vi "Test Periodic Timing.vi"() -> ()   [LabVIEW 2023, in "Volatus.lvlib" / "Module.lvclass"]
uses:
  Module.lvclass
  Module.lvclass/Module.ctl
panel:
  out "XY Graph":cluster{"elements":dbl[], "elements":dbl[]}(graph)
  out "Deadline":u32
  out "Message":string
  out "Periodic":bool
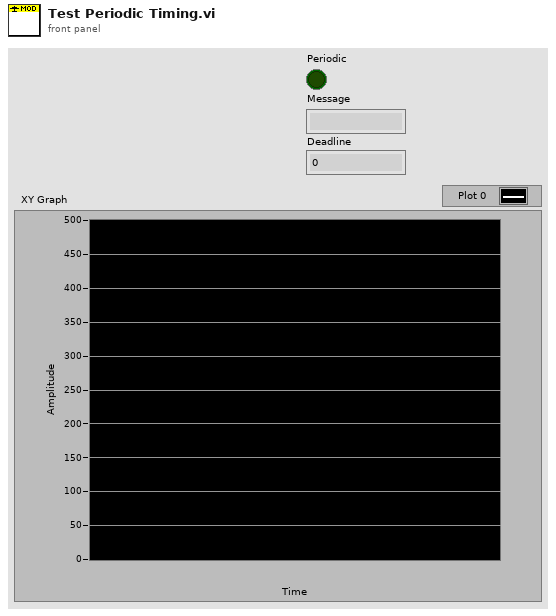
[diagram p1: front panel]
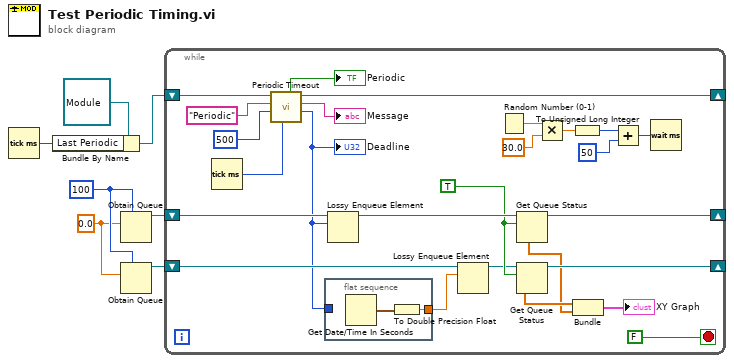
[diagram p0: block diagram]
diagram:
  w4 = 100 ("max queue size (-1, unlimited)")
  w3 = 0.0
  n1 = Tick Count (ms)() -> (millisecond timer value=w5:u32)
  n2 = Bundle By Name(cluster=refnum<class "Module.lvclass"> refnum ("Module in"), "Last Periodic"=w5) -> (w6:refnum<class "Module.lvclass">)
  n3 = Obtain Queue(max queue size (-1, unlimited)=w4, element data type=w3) -> (queue out=w2:refnum<queue>)  [unwired: 3 in, 2 out]
  n4 = Obtain Queue(max queue size (-1, unlimited)=w4, element data type=w3) -> (queue out=w1:refnum<queue>)  [unwired: 3 in, 2 out]
  n5 = while {
    shift-right: [w8] -> _
    shift-left: w6 -> [w29]
    shift-right: [w17] -> _
    shift-left: w1 -> [w18]
    shift-right: [w16] -> _
    shift-left: w2 -> [w20]
    stop <- FALSE stop-if-true
    w15 = TRUE ("return elements? (F)")
    n6 = Tick Count (ms)() -> (millisecond timer value=w27:u32)
    n7 = call "Periodic Timeout.vi"("Now"=w27, "Period/Timeout"=500, "Periodic Name"="Periodic", "Module in"=w29) -> ("Deadline"=w10:u32, "Message"=→"Message":string, "Module out"=w8:refnum<class "Module.lvclass">, "Periodic"=→"Periodic":bool)  [unwired: 4 in]
    "Deadline" <- w10
    n8 = flat-sequence {
      tunnel: w10 -> [_]
      tunnel: [w34] -> w9
      frame #0 {
        n9 = Get Date/Time In Seconds() -> (seconds since 1Jan1904=w35:timestamp)
        n10 = To Double Precision Float(number=w35) -> (double precision float=w34:dbl)
      }
    }
    n11 = Lossy Enqueue Element(queue=w20, element=w10) -> (queue out=w19:refnum<queue>)  [unwired: 1 in, 3 out]
    n12 = Lossy Enqueue Element(queue=w18, element=w9) -> (queue out=w11:refnum<queue>)  [unwired: 1 in, 3 out]
    n13 = Random Number (0-1)() -> (number: 0 to 1=w26:dbl)
    n14 = Get Queue Status(queue=w19, return elements? (F)=w15) -> (queue out=w16:refnum<queue>, elements=w13:dbl[])  [unwired: 1 in, 6 out]
    n15 = Get Queue Status(queue=w11, return elements? (F)=w15) -> (queue out=w17:refnum<queue>, elements=w14:dbl[])  [unwired: 1 in, 6 out]
    n16 = Multiply(x=w26, y=30.0) -> (x*y=w24:dbl)
    n17 = To Unsigned Long Integer(number=w24) -> (unsigned 32bit integer=w23:u32)
    n18 = Bundle("elements"=w14, "elements"=w13) -> (→"XY Graph":cluster{"elements":dbl[], "elements":dbl[]})  [unwired: 1 in]
    n19 = Add(x=w23, y=u32 50 ("milliseconds to wait")) -> (x+y=w21:u32)
    n20 = Wait (ms)(milliseconds to wait=w21) -> ()  [unwired: 1 out]
  }
